vi "sonic test.vi"   [LabVIEW 2016, in "Test2.lvrbt"]
uses:
  Test2.lvrbt
  <vilib>/NXT/Hardware/Plugins/Tetrix DC Motor/TetrixDCMotorAddress.ctl
  <vilib>/NXT/Block Support/NXT_InputPort.ctl
  <vilib>/NXT/NXTIO Xnodes/NXTIONodeSubVIs/TETRIX IO Move DC Motors.vi
  <vilib>/NXT/Dual Mode Library/Waits/Wait_EV3_Ultrasonic_Centimeter_Closer.vi
  <vilib>/NXT/NXTIO Xnodes/NXTIONodeSubVIs/TETRIX IO Stop DC Motors.vi
  <vilib>/NXT/Dual Mode Library/Waits/Wait_Num.vi
  <vilib>/NXT/Dual Mode Library/Waits/Wait_EV3_Ultrasonic_Centimeters_Further.vi
  <vilib>/NXT/Subs/LVHSConnector.ctl
  <vilib>/NXT/NXTIO Xnodes/AddressXNode/NXTIOAddress.xnode
  <vilib>/NXT/NXTIO Xnodes/NXTIOXNode/NXTIO.xnode
  <vilib>/NXT/LegoClasses/BrickReference/BrickReference.lvclass
types:
  T1 = typedef "TetrixDCMotorAddress.ctl" = i32
  T2 = cluster{"TetrixDCMotor":T1, "TetrixDCMotor 2":T1}
  T3 = typedef "NXT_InputPort.ctl" = u32
  T4 = typedef "LVHSConnector.ctl" = refnum<class "BrickReference.lvclass">
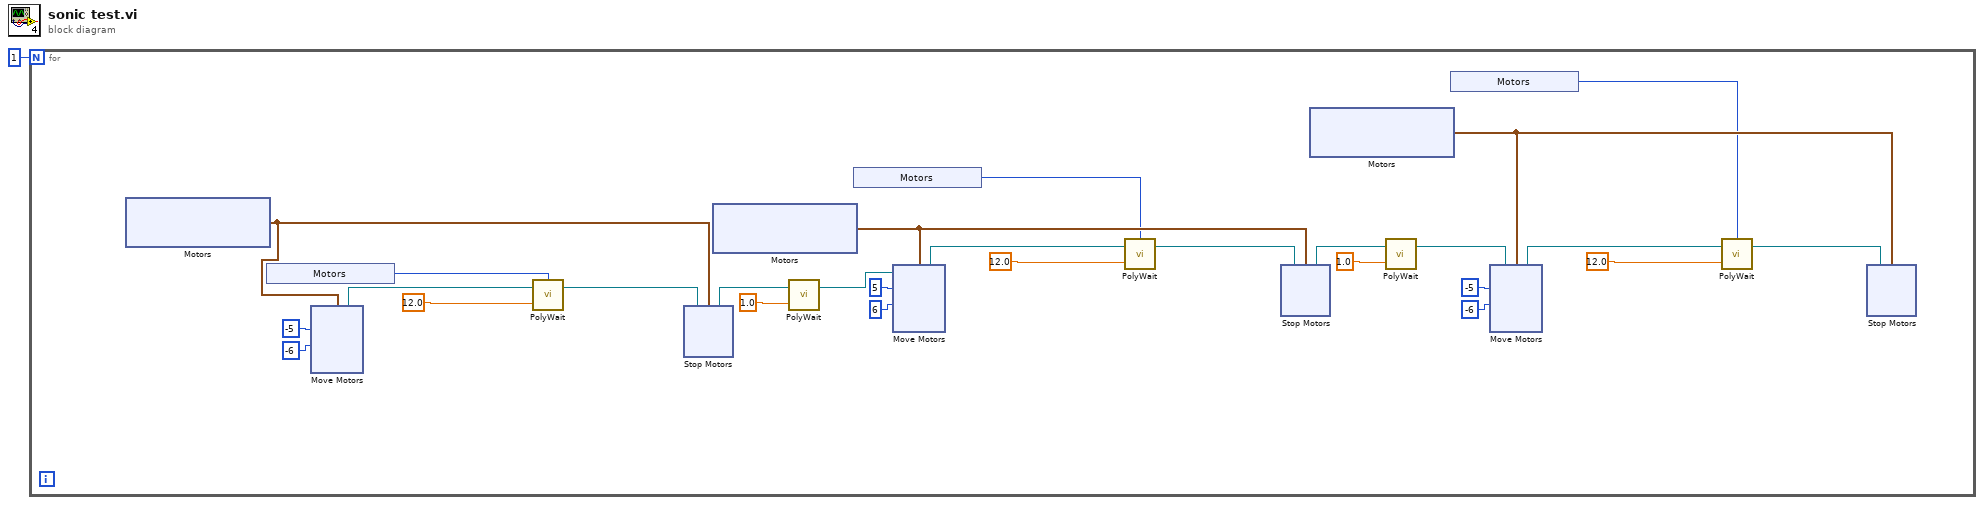
[diagram p0: block diagram]
diagram:
  n1 = for {
    N: 1 -> [_]
    n2 = xnode "Motors"() -> ("Motor"=w23:cluster{"TetrixDCMotor":T1, "TetrixDCMotor":T1})
    n3 = xnode "Motors"() -> ("Sensor"=w22:T3)
    n4 = xnode "Move Motors"("Power/Speed 2"=i8 -6, "Power/Speed 1"=i8 -5, "Motors"=w23) -> ("NXT/EV3"=w26:T4)  [unwired: 1 in]
    n5 = call-poly <vilib>:"PolyWait.vi"("Centimeters (40)"=sgl 12.0, "NXT/EV3"=w26, "Port (Port 1)"=w22) -> ("NXT/EV3"=w24:T4)  [unwired: 1 in]
    n6 = xnode "Stop Motors"("Motors"=w23, "NXT/EV3"=w24) -> ("NXT/EV3"=w21:T4)
    n7 = xnode "Motors"() -> ("Motor"=w14:cluster{"TetrixDCMotor":T1, "TetrixDCMotor":T1})
    n8 = call-poly <vilib>:"PolyWait.vi"("Time (1 sec)"=sgl 1.0, "NXT/EV3"=w21) -> ("NXT/EV3"=w12:T4)  [unwired: 2 in]
    n9 = xnode "Motors"() -> ("Sensor"=w13:T3)
    n10 = xnode "Move Motors"("Power/Speed 2"=i8 6, "Power/Speed 1"=i8 5, "Motors"=w14, "NXT/EV3"=w12) -> ("NXT/EV3"=w17:T4)
    n11 = call-poly <vilib>:"PolyWait.vi"("Centimeters (50)"=sgl 12.0 ("Centimeters (40)"), "NXT/EV3"=w17, "Port (Port 1)"=w13) -> ("NXT/EV3"=w15:T4)  [unwired: 1 in]
    n12 = xnode "Stop Motors"("Motors"=w14, "NXT/EV3"=w15) -> ("NXT/EV3"=w10:T4)
    n13 = xnode "Motors"() -> ("Motor"=w4:cluster{"TetrixDCMotor":T1, "TetrixDCMotor":T1})
    n14 = call-poly <vilib>:"PolyWait.vi"("Time (1 sec)"=sgl 1.0, "NXT/EV3"=w10) -> ("NXT/EV3"=w2:T4)  [unwired: 2 in]
    n15 = xnode "Motors"() -> ("Sensor"=w3:T3)
    n16 = xnode "Move Motors"("Power/Speed 2"=i8 -6, "Power/Speed 1"=i8 -5, "Motors"=w4, "NXT/EV3"=w2) -> ("NXT/EV3"=w7:T4)
    n17 = call-poly <vilib>:"PolyWait.vi"("Centimeters (40)"=sgl 12.0, "NXT/EV3"=w7, "Port (Port 1)"=w3) -> ("NXT/EV3"=w5:T4)  [unwired: 1 in]
    n18 = xnode "Stop Motors"("Motors"=w4, "NXT/EV3"=w5) -> ()  [unwired: 1 out]
  }
